vi "TubingCompensation.vi"(7 "NyquistLimitedCoefficients":dbl[](array[numeric]), 10 "mutedData":dbl[](array[numeric]), 11 "SamplingFreq":dbl) -> (2 "boostedData":dbl[](array[numeric]))   [LabVIEW 2011]
uses:
  <vilib>/Analysis/NI_AALBase.lvlib
panel:
  out "meanDifference":dbl format="%.2e"
  out "Waveform Graph":dbl[][](graph)
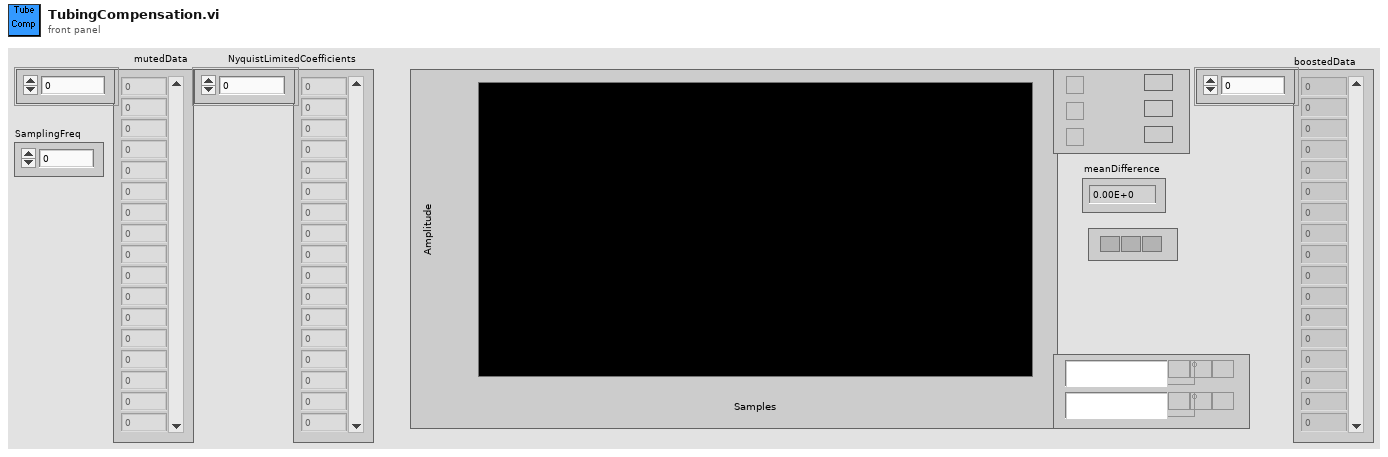
[diagram p1: front panel]
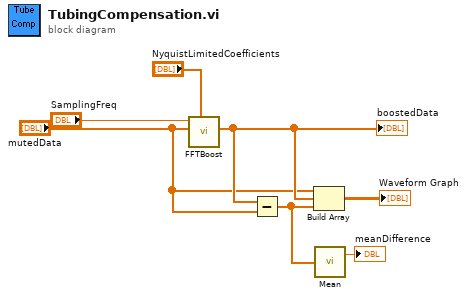
[diagram p0: block diagram]
diagram:
  n1 = call "FFTBoost.vi"("CompensationCoefficients"="NyquistLimitedCoefficients", "mutedData"="mutedData", "SamplingFreq (for graph)"="SamplingFreq") -> ("boostedData"=w6:dbl[])  [unwired: 8 out]
  "boostedData" <- w6
  n2 = Subtract(x=w6, y="mutedData") -> (x-y=w2:dbl[])
  n3 = Build Array("mutedData", w6, w2) -> (→"Waveform Graph":dbl[][])
  n4 = call <vilib>:"Mean.vi"("X"=w2) -> ("mean"=→"meanDifference":dbl)  [unwired: 1 out]
